vi "oa_TV Ptbypt Interpolation (1Chan).vi"(6 "buffer size":i32=4 min=1, 7 "reset? (F)":bool, 8 "error in (no error)":errorcluster, 9 "dX":dbl=0.0010714285714285715, 10 "Y":dbl[](array[numeric]), 11 "X":dbl[](array[numeric])) -> (0 "error out":errorcluster, 1 "X0":dbl, 2 "resampled X":dbl[](array[numeric]), 3 "resampled Y":dbl[](array[numeric]))   [LabVIEW 2017, in "SoundVib_Torsional.lvlib"]
uses:
  <vilib>/addons/Sound and Vibration/Order Analysis/Torsional Vibration/SoundVib_Torsional.lvlib
  <vilib>/Analysis/1siggen.llb/Ramp Pattern by Samples.vi
  <vilib>/Analysis/NI_AALBase.lvlib
  <vilib>/gmath/NI_Gmath.lvlib
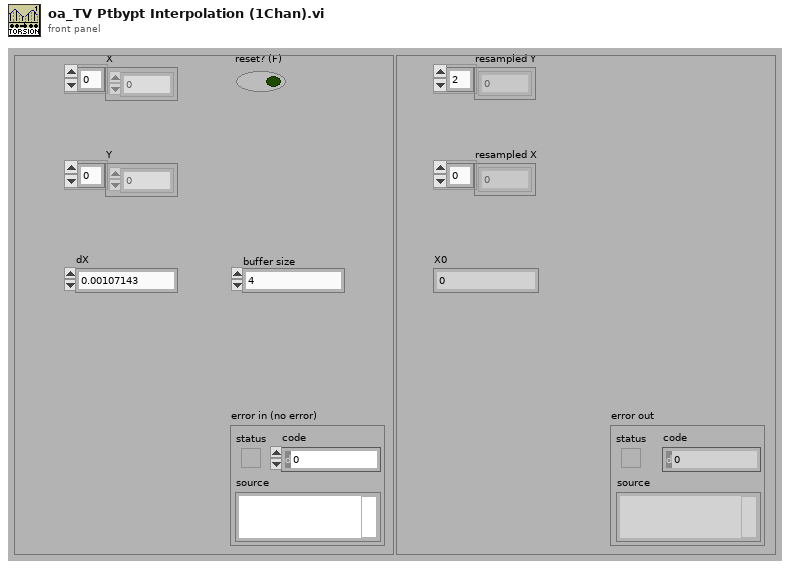
[diagram p1: front panel]
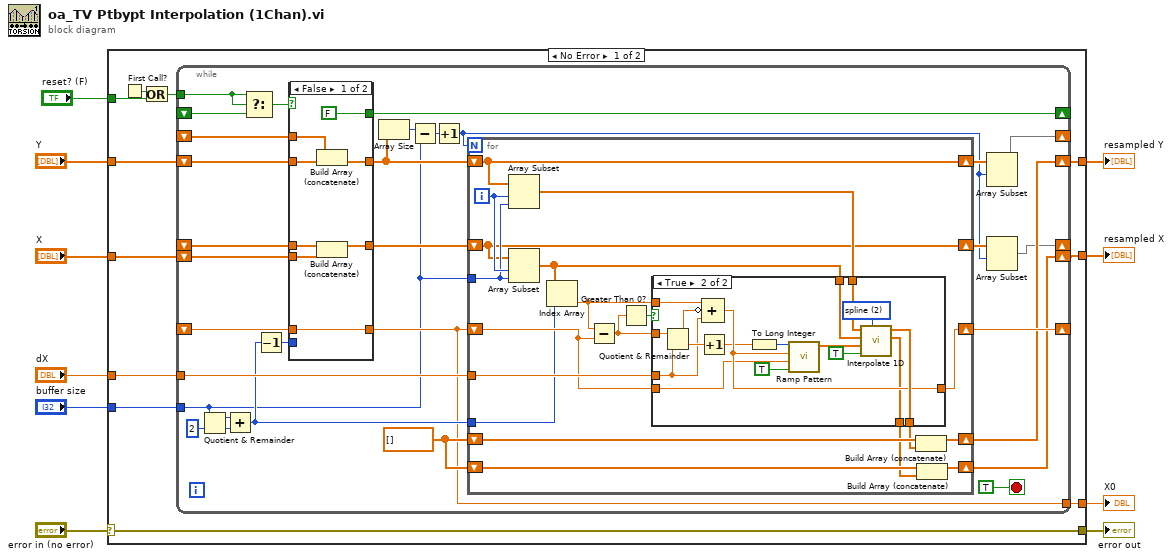
[diagram p0: block diagram]
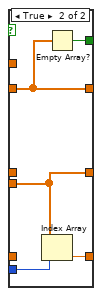
[diagram p2: hidden frame]
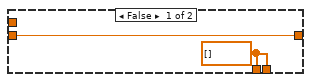
[diagram p3: hidden frame]
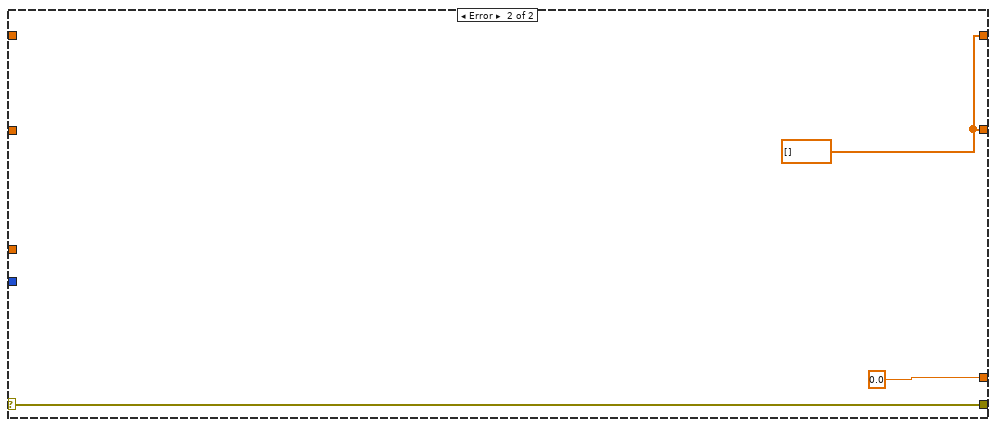
[diagram p4: hidden frame]
diagram:
  n1 = case shown="No Error" "error in (no error)" {
    selector: "error in (no error)" -> [w16 w106]
    tunnel: "buffer size" -> [w21 _]
    tunnel: "dX" -> [w20 _]
    tunnel: "reset? (F)" -> [w12 _]
    tunnel: "X" -> [w19 _]
    tunnel: "Y" -> [w18 _]
    tunnel: [w17 w104] -> w7
    tunnel: [w16 w106] -> w5
    tunnel: [w14 0.0 ("Numeric")] -> w4
    tunnel: [w13 w104] -> w3
    frame No Error {
      n2 = First Call?() -> (First Call?: T/F=w11:bool)
      n3 = Or(x=w11, y=w12) -> (x .or. y?=w15:bool)
      n4 = while {
        tunnel: w21 -> [w28]
        tunnel: w20 -> [w51]
        shift-right: [w50] -> _
        shift-left: _ -> [w34]
        tunnel: w15 -> [w47]
        shift-right: [w23] -> _
        shift-left: _ -> [w32]
        shift-right: [w27] -> _
        shift-left: _ -> [w33]
        tunnel: [w36] -> w14
        shift-right: [w35] -> _
        shift-left: _ -> [w46]
        shift-right: [w49] -> w17
        shift-left: w18 -> [w39]
        shift-right: [w48] -> w13
        shift-left: w19 -> [w38]
        stop <- TRUE stop-if-true
        w41 = dbl[] []
        n5 = Quotient & Remainder(x=w28, y=2) -> (x-y*floor(x/y)=w44:i32, floor(x/y)=w45:i32)
        n6 = Add(x=w44, y=w45) -> (x+y=w42:i32)
        n7 = Select(t=w47, s=w47, f=w46) -> (s? t:f=w40:bool)
        n8 = Decrement(x=w42) -> (x-1=w37:i32)
        n9 = case shown="False" w40 {
          tunnel: w39 -> [w57 w63]
          tunnel: w38 -> [w54 w62]
          tunnel: w37 -> [_ w64]
          tunnel: [w59 w61] -> w36
          tunnel: [w56 w63] -> w30
          tunnel: [w53 w62] -> w31
          tunnel: [FALSE ("empty?") w65] -> w35
          tunnel: w34 -> [w59 _]
          tunnel: w33 -> [w58 _]
          tunnel: w32 -> [w55 _]
          frame False {
            n10 = Build Array (concatenate)(w58, w57) -> (w56:dbl[])
            n11 = Build Array (concatenate)(w55, w54) -> (w53:dbl[])
          }
          frame True {
            n12 = Index Array(array=w62, index=w64) -> (element=w61:dbl)
            n13 = Empty Array?(array=w63) -> (empty?=w65:bool)
          }
        }
        n14 = Array Size(array=w30) -> (size(s)=w29:i32)
        n15 = Subtract(x=w29, y=w28) -> (x-y=w25:i32)
        n16 = Increment(x=w25) -> (x+1=w22:i32)
        n17 = for {
          N: w22 -> [_]
          shift-right: [w71] -> w26
          shift-left: w30 -> [w71]
          shift-right: [w66] -> w24
          shift-left: w31 -> [w66]
          shift-right: [w83] -> w50
          shift-left: w36 -> [w80]
          tunnel: w42 -> [w72]
          tunnel: w51 -> [w84]
          shift-right: [w76] -> w49
          shift-left: w41 -> [w82]
          shift-right: [w74] -> w48
          shift-left: w41 -> [w75]
          tunnel: w28 -> [w68]
          i -> [w69]
          n18 = Array Subset(array=w71, index=w69, length=w68) -> (w70:dbl[])
          n19 = Array Subset(array=w66, index=w69, length=w68) -> (w67:dbl[])
          n20 = Index Array(array=w67, index=w72) -> (element=w77:dbl)
          n21 = Subtract(x=w77, y=w80) -> (x-y=w79:dbl)
          n22 = Greater Than 0?(x=w79) -> (x > 0?=w78:bool)
          n23 = case shown="True" w78 {
            tunnel: w84 -> [_ w94]
            tunnel: [w86 w96] -> w83
            tunnel: [w85 w103] -> w81
            tunnel: w70 -> [_ w102]
            tunnel: w67 -> [_ w91]
            tunnel: w80 -> [w86 w95]
            tunnel: w79 -> [_ w101]
            tunnel: w77 -> [_ w99]
            tunnel: [w85 w89] -> w73
            frame False {
              w85 = dbl[] [] ("xi used")
            }
            frame True {
              w88 = 2 items=["nearest", "linear", "spline", "cubic Hermite", "Lagrange"] ("method")
              n24 = Quotient & Remainder(x=w101, y=w94) -> (x-y*floor(x/y)=w98:dbl, floor(x/y)=w100:dbl)
              n25 = Increment(x=w100) -> (x+1=w93:dbl)
              n26 = Compound Arithmetic op=ADD(w99, invert w98, w94) -> (w96:dbl)
              n27 = To Long Integer(number=w93) -> (32bit integer=w92:i32)
              n28 = call-poly <vilib>:"Ramp Pattern.vi"("exclude end?"=TRUE, "start"=w95, "end"=w96, "samples"=w92) -> ("Ramp Pattern"=w90:dbl[])  [unwired: 6 in, 1 out]
              n29 = call <vilib>:"Interpolate 1D.vi"("method"=w88, "X is monotonic"=TRUE, "xi"=w90, "X"=w91, "Y"=w102) -> ("xi used"=w89:dbl[], "yi"=w103:dbl[])  [unwired: 4 in, 1 out]
            }
          }
          n30 = Build Array (concatenate)(w82, w81) -> (w76:dbl[])
          n31 = Build Array (concatenate)(w75, w73) -> (w74:dbl[])
        }
        n32 = Array Subset(array=w26, index=w22) -> (w27:dbl[])  [unwired: 1 in]
        n33 = Array Subset(array=w24, index=w22) -> (w23:dbl[])  [unwired: 1 in]
      }
    }
    frame Error {
      w104 = dbl[] []
    }
  }
  "resampled Y" <- w7
  "error out" <- w5
  "X0" <- w4
  "resampled X" <- w3
